vi "Event Self.vi"(10 "Msg":refnum<class "Msg.lvclass">, 11 "Base Event Actor in":refnum<class "Base Event Actor.lvclass">) -> (3 "Base Event Actor out":refnum<class "Base Event Actor.lvclass">)   [LabVIEW 2021, in "jettl.lvlib" / "Base Event Actor.lvclass"]
uses:
  Base Event Actor.lvclass
  Msg/Msg/Msg.lvclass
  Base Event Actor.lvclass/Base Event Actor.ctl
  jettl.lvlib
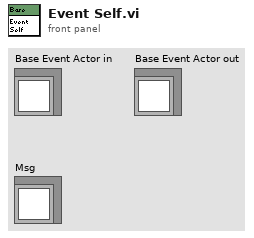
[diagram p1: front panel]
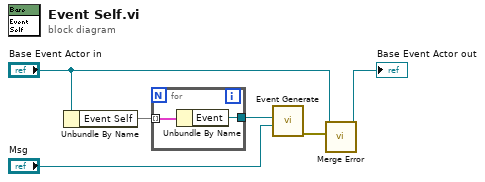
[diagram p0: block diagram]
diagram:
  n1 = Unbundle By Name("Base Event Actor in") -> ("Event Self"=w6:map{string, refnum<data-value>})
  n2 = for {
    tunnel: [w7] -> w3
    tunnel: w6 -> [w8] mode=indexing
    n3 = Unbundle By Name(w8) -> ("Event"=w7:refnum<data-value>)
  }
  n4 = call "Event Generate.vi"("Msg"="Msg", "Event"=w3) -> ("error out"=w2:errorcluster)  [unwired: 9 in]
  n5 = call-dynamic "Merge Error.vi"("Error"=w2, "Base Event Actor in"="Base Event Actor in") -> ("Base Event Actor out"=→"Base Event Actor out":refnum<class "Base Event Actor.lvclass">)  [unwired: 9 in]
